vi "GetPieceArray.vi"(8 "error in (no error)":errorcluster, 11 "object in":refnum<class "Board.lvclass">) -> (0 "error out":errorcluster, 2 "pieceArray":refnum<class "Piece.lvclass">[][](array[class]), 3 "object out":refnum<class "Board.lvclass">)   [LabVIEW 2020]
uses:
  Board.lvclass
  Pieces/Piece.lvclass
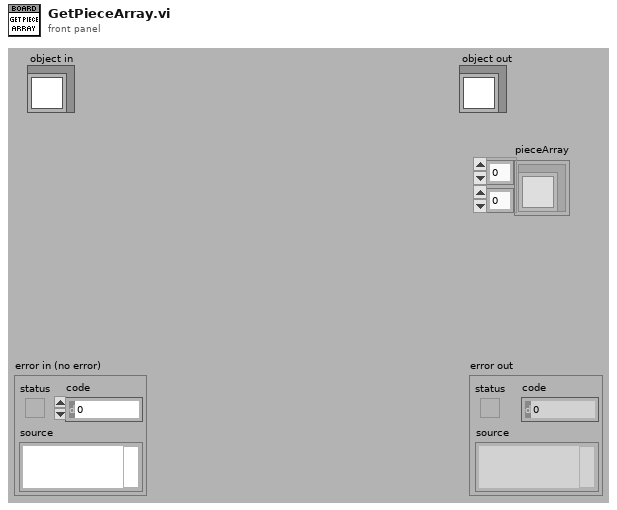
[diagram p1: front panel]
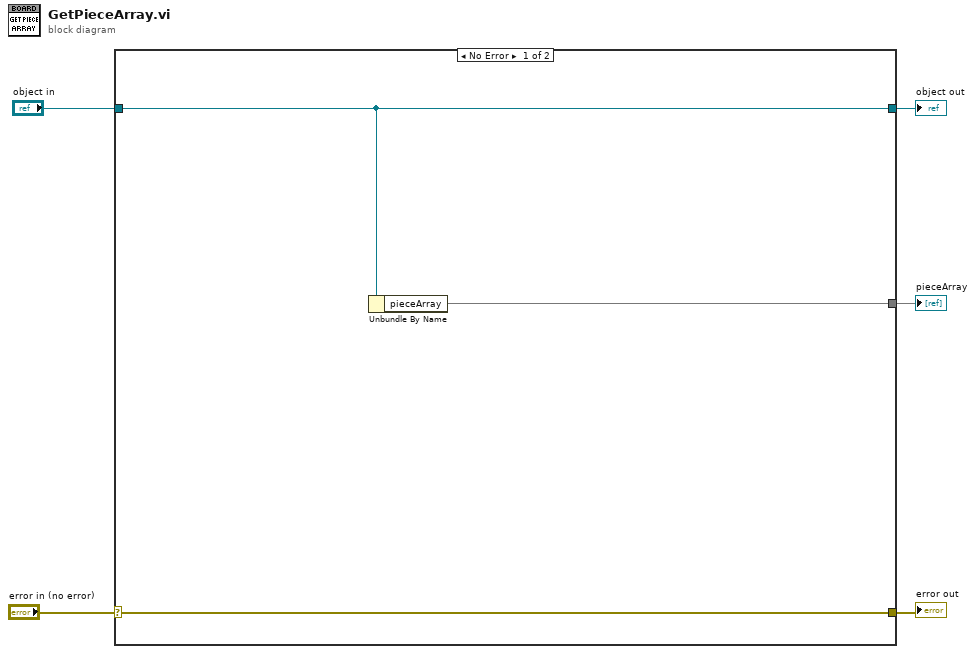
[diagram p0: block diagram]
diagram:
  n1 = case shown="No Error" "error in (no error)" {
    selector: "error in (no error)" -> [w7 w10]
    tunnel: [w7 w10] -> w4
    tunnel: [w6 w9] -> w2
    tunnel: "object in" -> [w6 w9]
    tunnel: [w8 _] -> w1
    frame No Error {
      n2 = Unbundle By Name(w6) -> ("pieceArray"=w8)
    }
    frame Error {
    }
  }
  "error out" <- w4
  "object out" <- w2
  "pieceArray" <- w1
